vi "Analog Write.vi"   [LabVIEW 2013, in "LVH-LINX.lvlib"]
uses:
  <vilib>/LabVIEW Hacker/LINX/LVH-LINX.lvlib
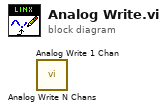
[diagram p0: block diagram]
diagram:
  n1 = call <vilib>:"Analog Write N Chans.vi"() -> ()  [unwired: 10 in, 2 out]
  n2 = call <vilib>:"Analog Write 1 Chan.vi"() -> ()  [unwired: 10 in, 2 out]
